vi "Cannon Get.vi"(1 "Throttle":dbl) -> ()   [LabVIEW 2012]
uses:
  Cannon Global Data.vi
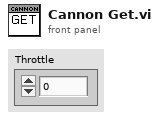
[diagram p1: front panel]
types:
  T1 = cluster{"Throttle":dbl, "RPM":dbl, "Motor VBus":dbl}
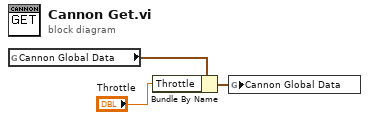
[diagram p0: block diagram]
diagram:
  n1 = global read "Cannon Global Data.vi" "Cannon Global Data"() -> (w2:T1)
  n2 = Bundle By Name(cluster=w2, "Throttle"="Throttle") -> (w3:T1)
  n3 = global write "Cannon Global Data.vi" "Cannon Global Data"(w3) -> ()
